vi "Publish Sample to Container.vi"(8 "error in (no error)":errorcluster, 10 "Containers":T1[](array[typedef]), 11 "Sample in":refnum<class "Sample.lvclass">) -> (0 "error out":errorcluster, 3 "Sample out":refnum<class "Sample.lvclass">)   [LabVIEW 2015, in "Sample.lvclass"]
uses:
  Sample.lvclass
  Controls/Sample Container.ctl
  Sample.lvclass/Sample.ctl
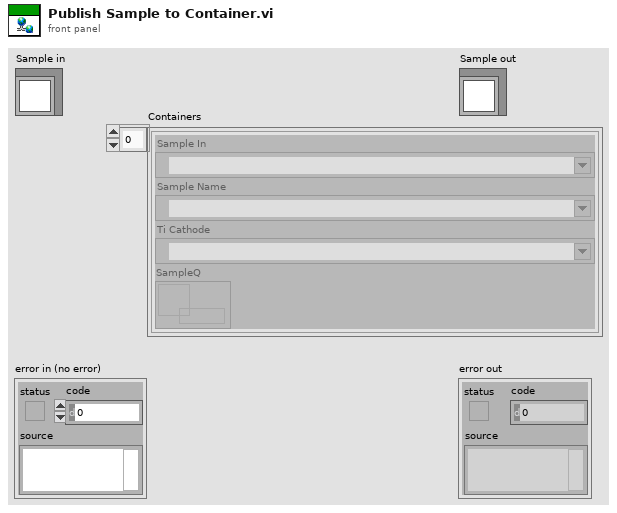
[diagram p1: front panel]
types:
  T1 = typedef "Sample Container.ctl" = cluster{"Sample In":refnum<k21>, "Sample Name":refnum<k21>, "Ti Cathode":refnum<k21>, "SampleQ":refnum<queue>}
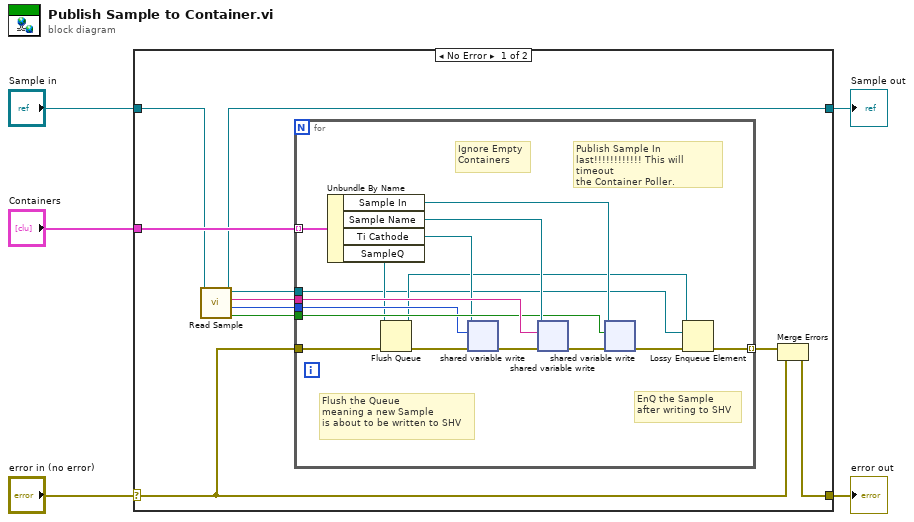
[diagram p0: block diagram]
diagram:
  n1 = case shown="No Error" "error in (no error)" {
    selector: "error in (no error)" -> [w6 w32]
    tunnel: [w7 w32] -> w4
    tunnel: [w9 w31] -> w2
    tunnel: "Sample in" -> [w10 w31]
    tunnel: "Containers" -> [w11 _]
    frame No Error {
      n2 = call "Read Sample.vi"("Sample in"=w10) -> ("Sample In"=w14:bool, "Ti Cathode"=w12:i8, "Name"=w13:string, "Sample out"=w9:refnum<class "Sample.lvclass">)  [unwired: 6 in, 1 out]
      n3 = for {
        tunnel: w11 -> [w24] mode=indexing
        tunnel: w6 -> [w19]
        tunnel: w14 -> [w25]
        tunnel: w13 -> [w26]
        tunnel: w12 -> [w22]
        tunnel: w9 -> [w15]
        tunnel: [w17] -> w8 mode=indexing
        # "EnQ the Sample\nafter writing to SHV"
        # "Flush the Queue\nmeaning a new Sample\nis about to be written to SHV"
        # "Publish Sample In\nlast!!!!!!!!!!!! This will timeout\nthe Container Poller."
        # "Ignore Empty\nContainers"
        n4 = Unbundle By Name(w24) -> ("Sample In"=w29:refnum<k21>, "Sample Name"=w30:refnum<k21>, "Ti Cathode"=w23:refnum<k21>, "SampleQ"=w20:refnum<queue>)
        n5 = Flush Queue(queue=w20, error in (no error)=w19) -> (queue out=w16:refnum<queue>, error out=w21:errorcluster)  [unwired: 1 out]
        n6 = shared-variable-write(w23, w21, w22) -> (w28:errorcluster)  [unwired: 1 out]
        n7 = shared-variable-write(w30, w28, w26) -> (w27:errorcluster)  [unwired: 1 out]
        n8 = shared-variable-write(w29, w27, w25) -> (w18:errorcluster)  [unwired: 1 out]
        n9 = Lossy Enqueue Element(queue=w16, element=w15, error in (no error)=w18) -> (error out=w17:errorcluster)  [unwired: 3 out]
      }
      n10 = Merge Errors(w8, w6) -> (w7:errorcluster)
    }
    frame Error {
    }
  }
  "error out" <- w4
  "Sample out" <- w2
